vi "Get Communication Specific Objects.vi"(8 "error in":errorcluster, 11 "EDS in":refnum<class "EDS.lvclass">) -> (0 "error out":errorcluster, 2 "Entries":refnum<class "OD Entry.lvclass">[](array[class]), 3 "EDS out":refnum<class "EDS.lvclass">)   [LabVIEW 2024, in "EDS.lvlib" / "EDS.lvclass"]
uses:
  EDS.lvclass
  OD Entry/OD Entry.lvclass
  EDS.lvclass/EDS.ctl
  Sorted Object Dictionary/Sorted Object Dictionary.lvclass
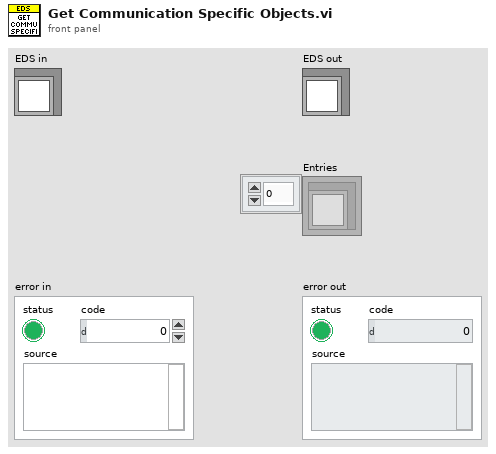
[diagram p1: front panel]
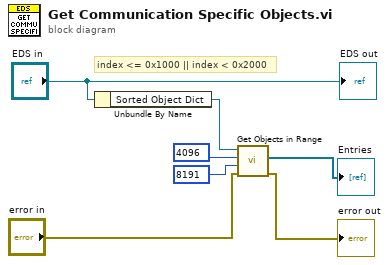
[diagram p0: block diagram]
diagram:
  # "index <= 0x1000 || index < 0x2000"
  n1 = Unbundle By Name("EDS in") -> ("Sorted Object Dict"=w6:refnum<class "Sorted Object Dictionary.lvclass">)
  n2 = call "Get Objects in Range.vi"("error in"="error in", "Upper Bound"=u16 8191 ("Lower Bound"), "Lower Bound"=u16 4096, "Sorted Object Dictionary in"=w6) -> ("error out"=→"error out":errorcluster, "Entries"=→"Entries":refnum<class "OD Entry.lvclass">[])  [unwired: 5 in, 1 out]
  "EDS out" <- "EDS in"
